vi "ISX3_Cmd_SetChannel.vi"(1 "Range Setting":u16(ring)=1 items=["100Ohm"=1, "10kOhm"=2, "1MOhm"=4], 2 "Measurement Channel":u8(ring)=1 items=["BNC"=1, "ExtensionPort"=2, "ExtensionPort2"=3]) -> (0 "set channel Cmd":u8[](array[numeric]))   [LabVIEW 2012, in "Sciospec ISX3 Impedance Analyzer.lvlib"]
uses:
  Sciospec ISX3 Impedance Analyzer.lvlib
panel:
  # "This VI generates the command to configure\nthe channel for the next measurement."
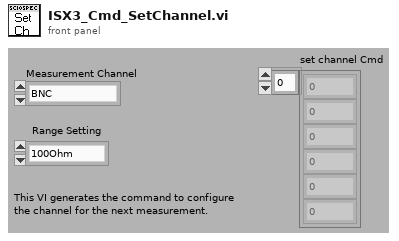
[diagram p1: front panel]
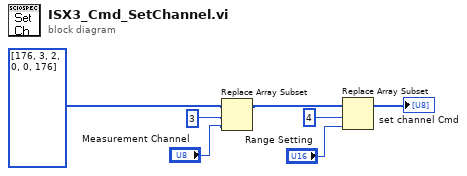
[diagram p0: block diagram]
diagram:
  n1 = Replace Array Subset(array=u8[] [176, 3, 2, 0, 0, 176], new element="Measurement Channel", index=3) -> (w4:u8[])
  n2 = Replace Array Subset(array=w4, new element="Range Setting", index=4) -> (→"set channel Cmd":u8[])
